vi "Create.vi"(8 "error in (no error)":errorcluster, 10 "Desired Stream Parameters":T1, 11 "Device ID":string) -> (0 "error out":errorcluster, 3 "New Stream":refnum<class "Stream.lvclass">)   [LabVIEW 2020, in "g_ar_toolkit.capture.lvlib" / "Stream.lvclass"]
uses:
  Stream.lvclass
  Stream Parameters.ctl
  Stream.lvclass/Stream.ctl
  g_ar_toolkit.common/g_ar_toolkit.common.lvlib
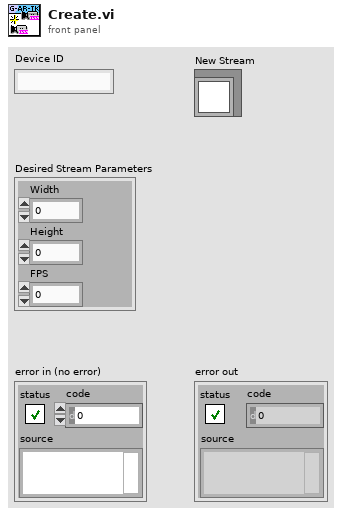
[diagram p1: front panel]
types:
  T1 = typedef "g_ar_toolkit.capture.lvlib/Stream.lvclass/Stream Parameters.ctl" = cluster{"Width":u16, "Height":u16, "FPS":u8}
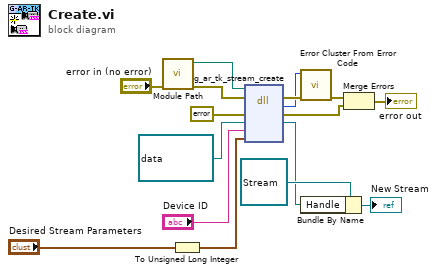
[diagram p0: block diagram]
diagram:
  n1 = call "Module Path.vi"("error in (no error)"="error in (no error)") -> ("error out"=w2:errorcluster, "Path"=w1:path)  [unwired: 9 in]
  n2 = To Unsigned Long Integer(number="Desired Stream Parameters") -> (unsigned 32bit integer=w8:cluster{"Width":u32, "Height":u32, "FPS":u32})
  n3 = dll-call lib="?" fn="g_ar_tk_stream_create" ("g_ar_toolkit.*.*:g_ar_tk_capture_stream_create")(path in=w1, error in=w2, "error_cluster"=errorcluster {"status"=FALSE, "code"=0, "source"=""} ("error constant"), "EDVR_strm"=refnum<data-value> refnum ("EDVR"), "device_id"="Device ID", "stream_type"=w8) -> (error out=w12:errorcluster, "MgErr"=w11:i32, "error_cluster"=w9:errorcluster, "EDVR_strm"=w6:refnum<data-value>)  [unwired: 3 in, 1 out]
  n4 = call <vilib>:"Error Cluster From Error Code.vi"("error in (no error)"=w12, "error code (0)"=w11) -> ("error out"=w10:errorcluster)  [unwired: 7 in]
  n5 = Bundle By Name(cluster=refnum<class "Stream.lvclass"> refnum ("g_ar_toolkit.capture.lvlib:Stream.lvclass"), "Handle"=w6) -> (→"New Stream":refnum<class "Stream.lvclass">)
  n6 = Merge Errors(w10, w9) -> (→"error out":errorcluster)
